vi "setVolume.vi"(8 "error in (no error)":errorcluster, 10 "volume":i32, 11 "Radio in":refnum<class "Radio.lvclass">) -> (0 "error out":errorcluster, 3 "Radio out":refnum<class "Radio.lvclass">)   [LabVIEW 2017, in "Radio.lvclass"]
uses:
  Radio.lvclass
  Radio.lvclass/Radio.ctl
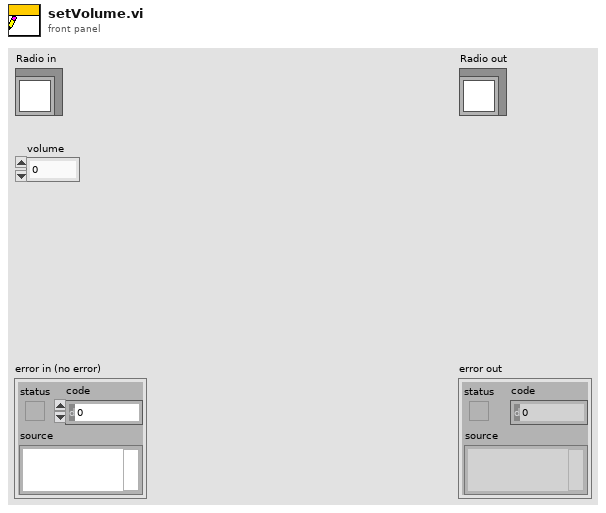
[diagram p1: front panel]
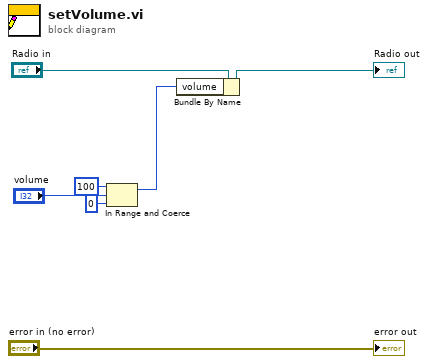
[diagram p0: block diagram]
diagram:
  n1 = In Range and Coerce(upper limit=100, x="volume", lower limit=0) -> (coerced(x)=w1:i32)  [unwired: 1 out]
  n2 = Bundle By Name(cluster="Radio in", "volume"=w1) -> (→"Radio out":refnum<class "Radio.lvclass">)
  "error out" <- "error in (no error)"
